vi "Get DVA Info wrapper.vi"(8 "error in (no error)":errorcluster caption="错误输入（无错误）", 9 "pDummyDvaInfo":T1, 10 "dwCanNodeId":u32, 11 "dwDevIndex":u32) -> (0 "error out":errorcluster caption="错误输出", 1 "pDummyDvaInfo out":T1, 3 "function return":u32)   [LabVIEW 2016, in "UISimCanFunc_wrapper.lvlib"]
doc: "_declspec (dllexport) DWORD GetDVAInfo_wrapper(DWORD dwDevIndex, DWORD dwCanNodeId, P_DUMMY_DVA_INFO_OBJ pDummyDvaInfo);"
uses:
  <userlib>/UISimCanFunc_wrapper/UISimCanFunc_wrapper.lvlib
  <userlib>/UISimCanFunc_wrapper/UISimCanFunc_wrapper.dll
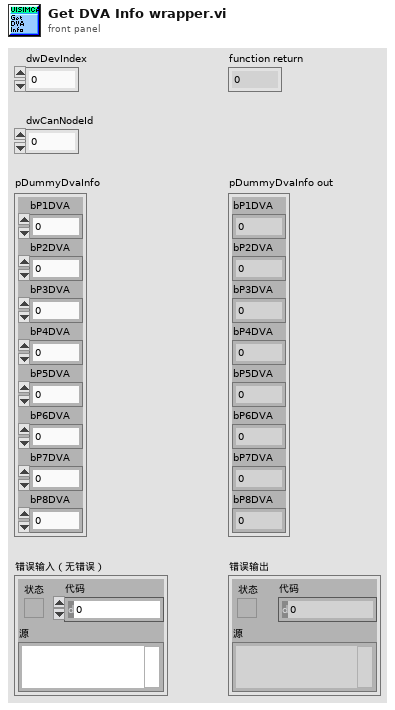
[diagram p1: front panel]
types:
  T1 = cluster{"bP1DVA":i32, "bP2DVA":i32, "bP3DVA":i32, "bP4DVA":i32, "bP5DVA":i32, "bP6DVA":i32, "bP7DVA":i32, "bP8DVA":i32}
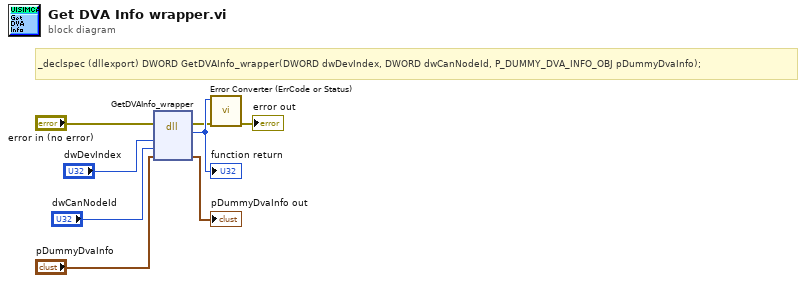
[diagram p0: block diagram]
diagram:
  # "_declspec (dllexport) DWORD GetDVAInfo_wrapper(DWORD dwDevIndex, DWORD dwCanNodeId, P_DUMMY_DVA_INFO_OBJ pDummyDvaInfo);"
  n1 = dll-call lib="C:/Program Files (x86)/National Instruments/LabVIEW 2016/user.lib/UISimCanFunc_wrapper/UISimCanFunc_wrapper.*" fn="GetDVAInfo_wrapper"(error in="error in (no error)", "dwDevIndex"="dwDevIndex", "dwCanNodeId"="dwCanNodeId", "pDummyDvaInfo"="pDummyDvaInfo") -> (error out=w2:errorcluster, w8:u32, "pDummyDvaInfo"=→"pDummyDvaInfo out":T1)  [unwired: 4 in, 1 out]
  "function return" <- w8
  n2 = call <userlib>:"Error Converter (ErrCode or Status).vi"("error in (no error)"=w2, "error code"=w8) -> ("error out"=→"error out":errorcluster)  [unwired: 9 in]
